vi "Force_Quit.vi"() -> ()   [LabVIEW 2011]
doc: "This VI allows the user to abort any VI currently in memory."
panel:
  in  "Exit":bool
  in  "Force Stop":bool
  in  "VI List":string(combo)
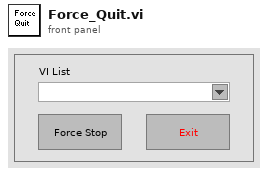
[diagram p1: front panel]
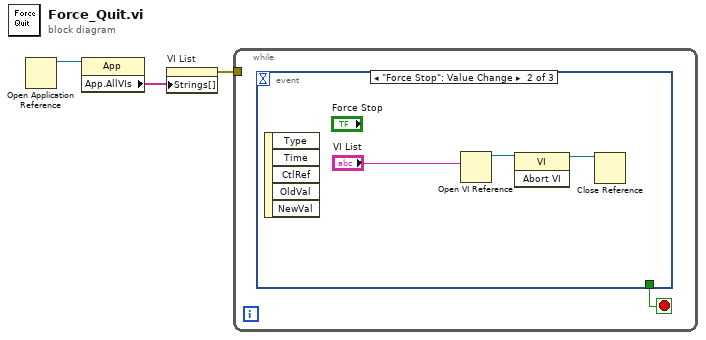
[diagram p0: block diagram]
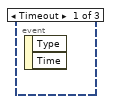
[diagram p2: hidden frame]
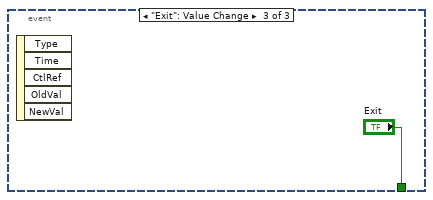
[diagram p3: hidden frame]
diagram:
  n1 = Open Application Reference() -> (3:w3:refnum<vi>)  [unwired: 4 in, 1 out]
  n2 = property class="App"(reference=w3) -> ("App.AllVIs"=w2:string[])  [unwired: 1 in, 2 out]
  n3 = property on="VI List" class="CmbBox"("Strings[]"=w2) -> (error out=w1:errorcluster)  [unwired: 2 in, 1 out]
  n4 = while {
    tunnel: w1 -> [_]
    stop <- w4 stop-if-true
    n5 = event shown="[1] \"Force Stop\": Value Change" {
      selector: _ -> [_ _ _]
      dyn-events: _ -> [_ _ _]
      timeout: _ -> [_ _ _]
      tunnel: [_ _ "Exit"] -> w4
      event Timeout {
        n6 = event-data() -> ()  [unwired: 1 in, 2 out]
      }
      event "Force Stop": Value Change {
        n7 = event-data() -> ()  [unwired: 1 in, 5 out]
        n8 = Open VI Reference(vi path="VI List") -> (vi reference=w6:refnum<vi>)  [unwired: 5 in, 1 out]
        n9 = invoke class="VI" method="Abort VI"(reference=w6) -> (reference out=w5:refnum<vi>)  [unwired: 2 in, 2 out]
        n10 = Close Reference(reference=w5) -> ()  [unwired: 1 in, 1 out]
      }
      event "Exit": Value Change {
        n11 = event-data() -> ()  [unwired: 1 in, 5 out]
      }
    }
  }
